vi "LV_UDP_client.vi"() -> ()   [LabVIEW 2020]
panel:
  in  "Send Test Image":bool
  in  "h":i32=10 min=1 max=5000 step=1
  in  "w":i32=1 min=1 max=5000 step=1
  out "Elaps ms":u32
  in  "Send Image":bool
  out "Path to Python script":path
  in  "Stop":bool
  out "Answer":string
  in  "Ping":bool
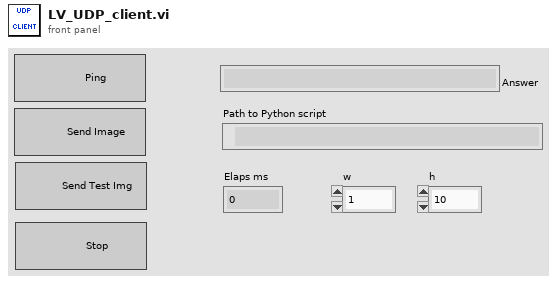
[diagram p1: front panel]
types:
  T1 = typedef "Image Type" = u32
  T2 = enum8{"Enabled", "Disabled", "Disabled and Grayed Out"}
  T3 = typedef "IMAQ Image.ctl" = refnum<image>
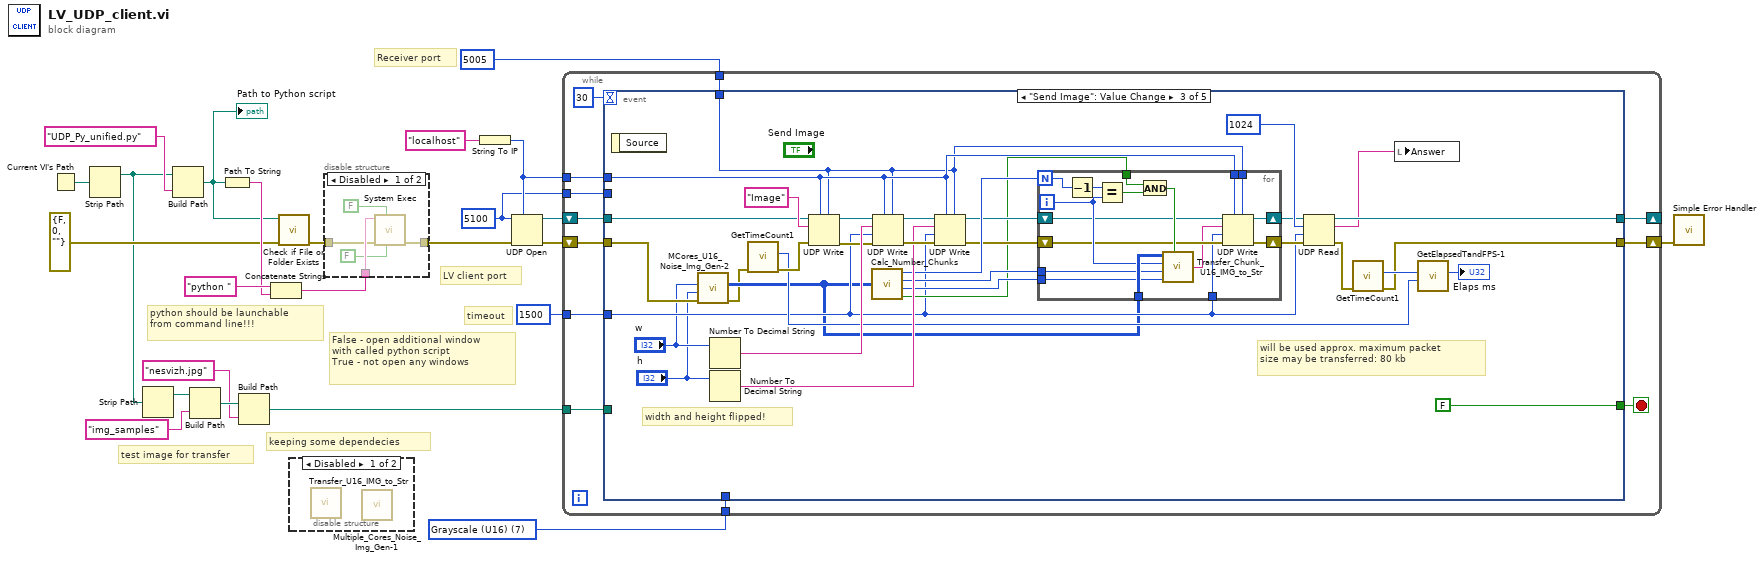
[diagram p0: block diagram]
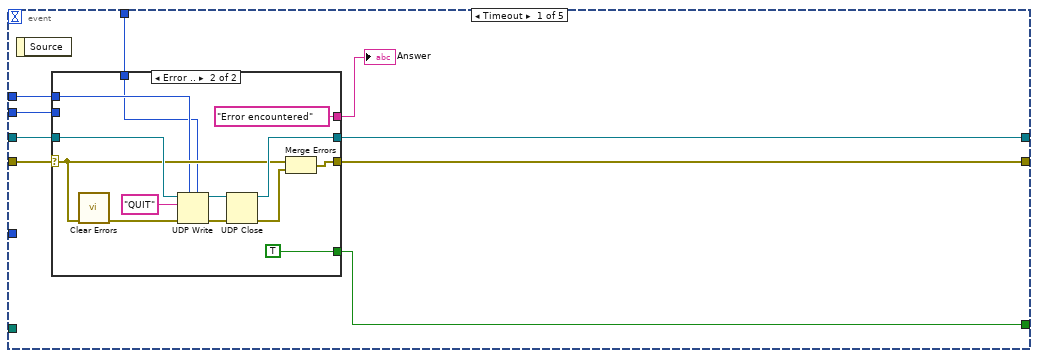
[diagram p4: hidden frame]
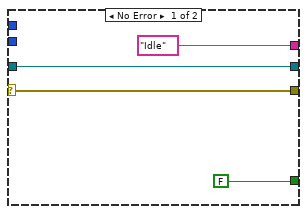
[diagram p5: hidden frame]
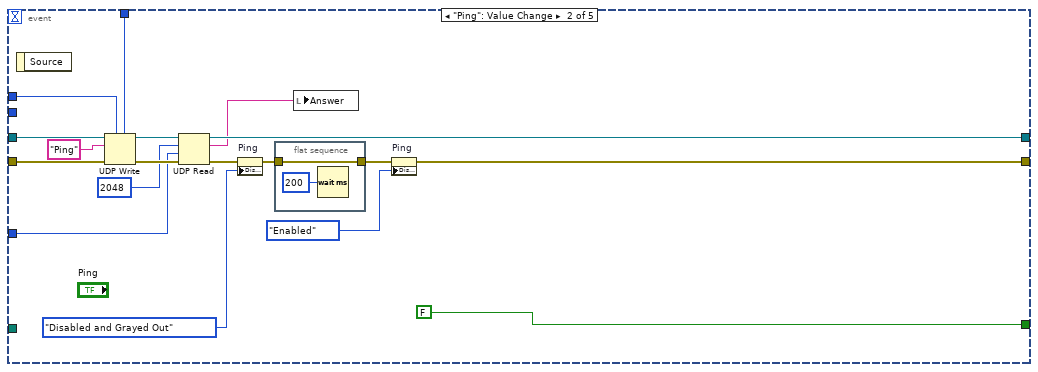
[diagram p6: hidden frame]
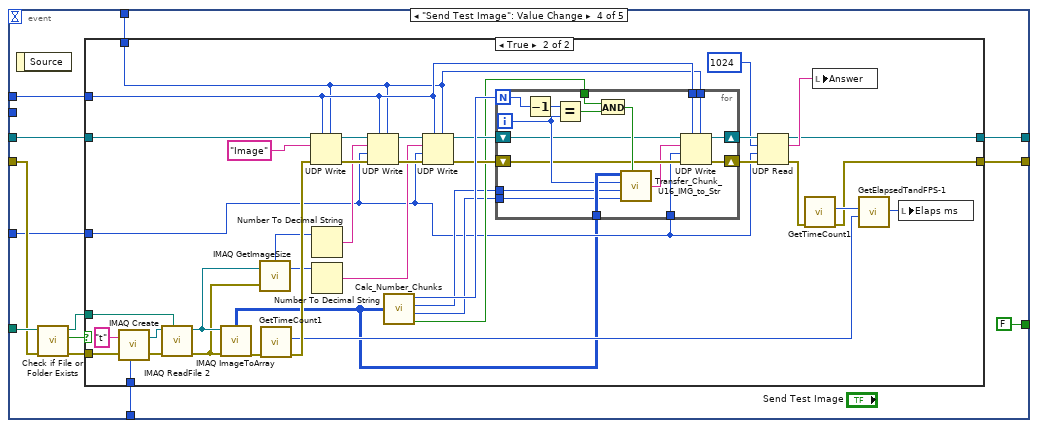
[diagram p7: hidden frame]
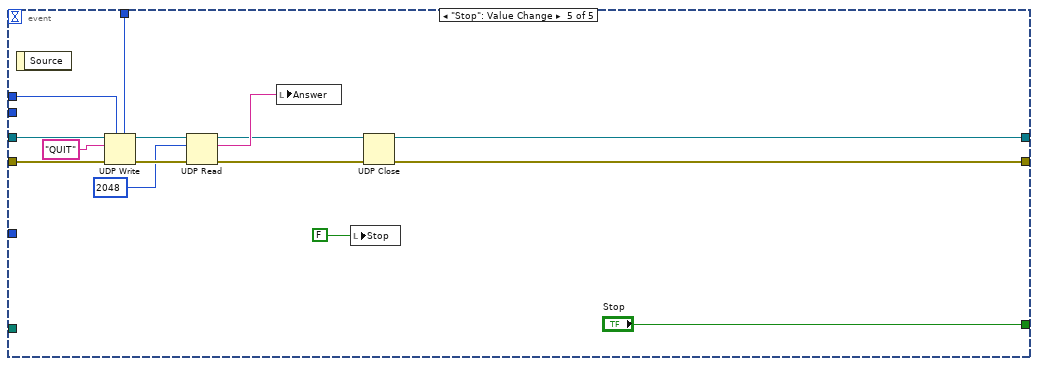
[diagram p9: hidden frame]
diagram:
  w1 = T1 7 items=["Grayscale (U8)", "Grayscale (I16)", "Grayscale (SGL)", "Complex (CSG)", "RGB (U32)", "HSL (U32)", "RGB (U64)", "Grayscale (U16)"] ("Image Type")
  w10 = u16 5100 ("remote port or service name")
  # "test image for transfer"
  # "keeping some dependecies"
  # "timeout"
  # "Receiver port"
  # "LV client port"
  # "False - open additional window\nwith called python script\nTrue - not open any windows"
  # "python should be launchable \nfrom command line!!!"
  n1 = Current VI's Path() -> (path=w23:path)
  n2 = Strip Path(path=w23) -> (stripped path=w7:path)  [unwired: 1 out]
  n3 = Strip Path(path=w7) -> (stripped path=w6:path)  [unwired: 1 out]
  n4 = Build Path(base path=w7, name or relative path="UDP_Py_unified.py" ("string")) -> (appended path=w17:path)
  "Path to Python script" <- w17
  n5 = Build Path(base path=w6, name or relative path="img_samples" ("string")) -> (appended path=w4:path)
  n6 = Path To String(path=w17) -> (string=w19:string)
  n7 = Build Path(base path=w4, name or relative path="nesvizh.jpg" ("string")) -> (appended path=w2:path)
  n8 = Concatenate Strings("python " ("command line"), w19) -> (w21:string)
  n9 = call <vilib>:"Check if File or Folder Exists.vi"("error in (no error)"=errorcluster {"status"=FALSE, "code"=0, "source"=""}, "path"=w17) -> ("error out"=w16:errorcluster)  [unwired: 7 in, 2 out]
  n10 = disable-structure shown="Disabled" {
    frame Disabled {
      n11 = call "Transfer_U16_IMG_to_Str.vi"() -> ()  [unwired: 1 in, 1 out]
      n12 = call "Multiple_Cores_Noise_Img_Gen-1.vi"() -> ()  [unwired: 10 in, 2 out]
    }
    frame Enabled {
    }
  }
  n13 = disable-structure shown="Disabled" {
    disable-tunnel: w21 -> [w29 _]
    disable-tunnel: [w28 w30] -> w15
    disable-tunnel: w16 -> [w26 w30]
    frame Disabled {
      n14 = call <vilib>:"System Exec.vi"("run minimized? (F)"=FALSE, "wait until completion? (T)"=FALSE, "error in (no error)"=w26, "command line"=w29) -> ("error out"=w28:errorcluster)  [unwired: 4 in, 3 out]
    }
    frame Enabled {
    }
  }
  n15 = String To IP(1:"localhost" ("address")) -> (0:w11:u32)
  n16 = UDP Open(7:w11, 8:w15, 11:w10) -> (port=w13:refnum<k16>, 0:w14:errorcluster)  [unwired: 2 in, 1 out]
  n17 = while {
    shift-right: [w39] -> _
    shift-left: w13 -> [w40]
    shift-right: [w37] -> w24
    shift-left: w14 -> [w41]
    tunnel: w11 -> [w35]
    tunnel: w10 -> [w36]
    tunnel: u16 5005 ("remote port or service name") -> [w34]
    tunnel: 1500 -> [w33]
    tunnel: w2 -> [w32]
    tunnel: w1 -> [w31]
    stop <- w38 stop-if-true
    n18 = event shown="[2] \"Send Image\": Value Change" {
      selector: _ -> [_ _ _ _ _]
      dyn-events: _ -> [_ _ _ _ _]
      timeout: 30 -> [_ _ _ _ _]
      tunnel: [w47 FALSE ("Stop") FALSE ("Stop") FALSE ("Stop") "Stop"] -> w38
      tunnel: w41 -> [w51 w80 w93 w150 w221]
      tunnel: w40 -> [w50 w79 w121 w145 w222]
      tunnel: [w49 w75 w115 w140 w223] -> w39
      tunnel: [w48 w82 w106 w141 w224] -> w37
      tunnel: w36 -> [w45 _ _ _ _]
      tunnel: w35 -> [w44 w71 w95 w144 w213]
      tunnel: w34 -> [w43 w70 w94 w143 w212]
      tunnel: w33 -> [_ w69 w96 w142 _]
      tunnel: w32 -> [_ _ _ w151 _]
      tunnel: w31 -> [_ _ _ w146 _]
      event Timeout {
        n19 = event-data() -> ()  [unwired: 1 in, 1 out]
        n20 = case shown="Error .." w51 {
          selector: w51 -> [w54 w59]
          tunnel: [w55 w66] -> w49
          tunnel: w50 -> [w55 w65]
          tunnel: [w54 w60] -> w48
          tunnel: [FALSE ("Stop") TRUE ("Stop")] -> w47
          tunnel: ["Idle" ("Answer") "Error encountered" ("Answer")] -> w46
          tunnel: w45 -> [_ _]
          tunnel: w44 -> [_ w57]
          tunnel: w43 -> [_ w56]
          frame No Error {
          }
          frame Error {
            n21 = call <vilib>:"Clear Errors.vi"("error in (no error)"=w59) -> ("error out"=w64:errorcluster)  [unwired: 5 in, 1 out]
            n22 = UDP Write(address=w57, port or service name=w56, connection ID=w65, data in="QUIT", 8:w64) -> (error out=w63:errorcluster, 3:w61:refnum<k16>)  [unwired: 1 in]
            n23 = UDP Close(connection ID=w61, 8:w63) -> (connection ID out=w66:refnum<k16>, error out=w58:errorcluster)
            n24 = Merge Errors(w59, w58) -> (w60:errorcluster)
          }
        }
        "Answer" <- w46
      }
      event "Ping": Value Change {
        n25 = event-data() -> ()  [unwired: 1 in, 1 out]
        n26 = UDP Write(address=w71, port or service name=w70, connection ID=w79, data in="Ping", 8:w80) -> (error out=w77:errorcluster, 3:w76:refnum<k16>)  [unwired: 1 in]
        n27 = UDP Read(connection ID=w76, max size (548)=2048 ("bytes to read"), timeout ms (25000)=w69, 8:w77) -> (data out=w72:string, error out=w74:errorcluster, 3:w75:refnum<k16>)  [unwired: 2 out]
        n28 = property on="Ping" class="Bool"(error in=w74, "DisabledEnum"=T2."Disabled and Grayed Out" ("Disabled")) -> (error out=w85:errorcluster)  [unwired: 1 in, 1 out]
        n29 = flat-sequence {
          tunnel: w85 -> [w87]
          tunnel: [w87] -> w83
          frame #0 {
            n30 = Wait (ms)(milliseconds to wait=u32 200) -> ()  [unwired: 1 out]
          }
        }
        n31 = local write "Answer"(w72) -> ()
        n32 = property on="Ping" class="Bool"(error in=w83, "DisabledEnum"=T2."Enabled" ("Disabled")) -> (error out=w82:errorcluster)  [unwired: 1 in, 1 out]
      }
      event "Send Image": Value Change {
        # "width and height flipped!"
        # "will be used approx. maximum packet \nsize may be transferred: 80 kb"
        n33 = event-data() -> ()  [unwired: 1 in, 1 out]
        n34 = call "MCores_U16_Noise_Img_Gen-2.vi"("error IN"=w93, "[IN] Width"="h", "[IN] Height"="w") -> ("error OUT"=w91:errorcluster, "[OUT] U16 Pixel Img"=w92:u16[][])  [unwired: 7 in]
        n35 = Number To Decimal String(number="w") -> (decimal integer string=w117:string)  [unwired: 1 in]
        n36 = Number To Decimal String(number="h") -> (decimal integer string=w113:string)  [unwired: 1 in]
        n37 = call "GetTimeCount1.vi"("error IN"=w91) -> ("error OUT"=w110:errorcluster, "[OUT] Timer Count"=w107:u32)  [unwired: 9 in]
        n38 = UDP Write(address=w95, port or service name=w94, connection ID=w121, data in="Image", 8:w110) -> (error out=w111:errorcluster, 3:w112:refnum<k16>)  [unwired: 1 in]
        n39 = call "Calc_Number_Chunks.vi"("[IN] U16 Pixel Img"=w92) -> ("[OUT] Number of chunks"=w103:i32, "[OUT] # rows single transfer"=w102:i32, "[OUT] # rows last transfer"=w101:i32, "[OUT] Not-equal last transfer"=w97:bool)
        n40 = UDP Write(address=w95, port or service name=w94, connection ID=w112, data in=w117, 8:w111, 9:w96) -> (error out=w120:errorcluster, 3:w119:refnum<k16>)
        n41 = UDP Write(address=w95, port or service name=w94, connection ID=w119, data in=w113, 8:w120, 9:w96) -> (error out=w99:errorcluster, 3:w100:refnum<k16>)
        n42 = for {
          N: w103 -> [w139]
          shift-right: [w129] -> w104
          shift-left: w99 -> [w130]
          tunnel: w92 -> [w137]
          tunnel: w102 -> [w132]
          tunnel: w101 -> [w131]
          shift-right: [w128] -> w98
          shift-left: w100 -> [w127]
          tunnel: w97 -> [w134]
          tunnel: w96 -> [w125]
          tunnel: w95 -> [w124]
          tunnel: w94 -> [w123]
          i -> [w135]
          n43 = Decrement(x=w139) -> (x-1=w138:i32)
          n44 = Equal?(x=w138, y=w135) -> (x = y?=w133:bool)
          n45 = And(x=w134, y=w133) -> (x .and. y?=w136:bool)
          n46 = call "Transfer_Chunk_U16_IMG_to_Str.vi"("[IN] U16 Pixel Img"=w137, "[IN] # of chunk"=w135, "[IN] # rows single transfer"=w132, "[IN] # rows last transfer"=w131, "[IN] Use remained rows"=w136) -> ("[OUT] Converted String"=w126:string)
          n47 = UDP Write(address=w124, port or service name=w123, connection ID=w127, data in=w126, 8:w130, 9:w125) -> (error out=w129:errorcluster, 3:w128:refnum<k16>)
        }
        n48 = UDP Read(connection ID=w98, max size (548)=1024 ("bytes to read"), timeout ms (25000)=w96, 8:w104) -> (data out=w114:string, error out=w109:errorcluster, 3:w115:refnum<k16>)  [unwired: 2 out]
        n49 = call "GetTimeCount1.vi"("error IN"=w109) -> ("error OUT"=w106:errorcluster, "[OUT] Timer Count"=w108:u32)  [unwired: 9 in]
        n50 = local write "Answer"(w114) -> ()
        n51 = call "GetElapsedTandFPS-1.vi"("[IN] Timer Count Before ALL [ms]"=w107, "[IN] Timer Count After ALL [ms]"=w108) -> ("[OUT] Elapsed time [ms]"=→"Elaps ms":u32)  [unwired: 3 in, 2 out]
      }
      event "Send Test Image": Value Change {
        n52 = event-data() -> ()  [unwired: 1 in, 1 out]
        n53 = call <vilib>:"Check if File or Folder Exists.vi"("error in (no error)"=w150, "path"=w151) -> ("error out"=w149:errorcluster, "file or folder exists?"=w148:bool, "dup path"=w147:path)  [unwired: 7 in]
        n54 = case shown="True" w148 {
          tunnel: w149 -> [w153 w194]
          tunnel: w147 -> [_ w189]
          tunnel: w146 -> [_ w193]
          tunnel: w145 -> [w154 w187]
          tunnel: w144 -> [_ w168]
          tunnel: w143 -> [_ w167]
          tunnel: w142 -> [_ w164]
          tunnel: [w153 w157] -> w141
          tunnel: [w154 w156] -> w140
          frame False {
          }
          frame True {
            n55 = call "IMAQ Create"("Image Name"="t", "Image Type"=w193, "error in (no error)"=w194) -> ("New Image"=w190:T3, "error out"=w191:errorcluster)  [unwired: 2 in]
            n56 = call "IMAQ ReadFile 2"("File Path"=w189, "error in (no error)"=w191, "Image"=w190) -> ("error out"=w183:errorcluster, "Image Out"=w184:T3)  [unwired: 4 in, 3 out]
            n57 = call "IMAQ ImageToArray"("error in (no error)"=w183, "Image"=w184) -> ("error out"=w188:errorcluster, "Image Pixels (U8)"=w155:u8[][])  [unwired: 2 in, 3 out]
            n58 = call "IMAQ GetImageSize"("Image"=w184, "error in (no error)"=w183) -> ("Y Resolution"=w181:i32, "X Resolution"=w182:i32)  [unwired: 2 in, 1 out]
            n59 = call "GetTimeCount1.vi"("error IN"=w188) -> ("error OUT"=w186:errorcluster, "[OUT] Timer Count"=w160:u32)  [unwired: 9 in]
            n60 = UDP Write(address=w168, port or service name=w167, connection ID=w187, data in="Image", 8:w186) -> (error out=w180:errorcluster, 3:w179:refnum<k16>)  [unwired: 1 in]
            n61 = Number To Decimal String(number=w182) -> (decimal integer string=w178:string)  [unwired: 1 in]
            n62 = Number To Decimal String(number=w181) -> (decimal integer string=w175:string)  [unwired: 1 in]
            n63 = UDP Write(address=w168, port or service name=w167, connection ID=w179, data in=w178, 8:w180, 9:w164) -> (error out=w176:errorcluster, 3:w177:refnum<k16>)
            n64 = call "Calc_Number_Chunks.vi"("[IN] U16 Pixel Img"=w155) -> ("[OUT] Number of chunks"=w174:i32, "[OUT] # rows single transfer"=w170:i32, "[OUT] # rows last transfer"=w169:i32, "[OUT] Not-equal last transfer"=w171:bool)
            n65 = UDP Write(address=w168, port or service name=w167, connection ID=w177, data in=w175, 8:w176, 9:w164) -> (error out=w172:errorcluster, 3:w173:refnum<k16>)
            n66 = for {
              N: w174 -> [w211]
              shift-right: [w201] -> w166
              shift-left: w172 -> [w202]
              tunnel: w155 -> [w209]
              tunnel: w170 -> [w204]
              tunnel: w169 -> [w203]
              shift-right: [w200] -> w165
              shift-left: w173 -> [w199]
              tunnel: w171 -> [w206]
              tunnel: w164 -> [w197]
              tunnel: w168 -> [w196]
              tunnel: w167 -> [w195]
              i -> [w207]
              n67 = Decrement(x=w211) -> (x-1=w210:i32)
              n68 = Equal?(x=w210, y=w207) -> (x = y?=w205:bool)
              n69 = And(x=w206, y=w205) -> (x .and. y?=w208:bool)
              n70 = call "Transfer_Chunk_U16_IMG_to_Str.vi"("[IN] U16 Pixel Img"=w209, "[IN] # of chunk"=w207, "[IN] # rows single transfer"=w204, "[IN] # rows last transfer"=w203, "[IN] Use remained rows"=w208) -> ("[OUT] Converted String"=w198:string)
              n71 = UDP Write(address=w196, port or service name=w195, connection ID=w199, data in=w198, 8:w202, 9:w197) -> (error out=w201:errorcluster, 3:w200:refnum<k16>)
            }
            n72 = UDP Read(connection ID=w165, max size (548)=1024 ("bytes to read"), timeout ms (25000)=w164, 8:w166) -> (data out=w163:string, error out=w162:errorcluster, 3:w156:refnum<k16>)  [unwired: 2 out]
            n73 = call "GetTimeCount1.vi"("error IN"=w162) -> ("error OUT"=w157:errorcluster, "[OUT] Timer Count"=w161:u32)  [unwired: 9 in]
            n74 = local write "Answer"(w163) -> ()
            n75 = call "GetElapsedTandFPS-1.vi"("[IN] Timer Count Before ALL [ms]"=w160, "[IN] Timer Count After ALL [ms]"=w161) -> ("[OUT] Elapsed time [ms]"=w158:u32)  [unwired: 3 in, 2 out]
            n76 = local write "Elaps ms"(w158) -> ()
          }
        }
      }
      event "Stop": Value Change {
        n77 = event-data() -> ()  [unwired: 1 in, 1 out]
        n78 = UDP Write(address=w213, port or service name=w212, connection ID=w222, data in="QUIT", 8:w221) -> (error out=w218:errorcluster, 3:w219:refnum<k16>)  [unwired: 1 in]
        n79 = UDP Read(connection ID=w219, max size (548)=2048 ("bytes to read"), 8:w218) -> (data out=w216:string, error out=w217:errorcluster, 3:w215:refnum<k16>)  [unwired: 1 in, 2 out]
        n80 = local write "Answer"(w216) -> ()
        n81 = local write "Stop"(FALSE ("Stop")) -> ()
        n82 = UDP Close(connection ID=w215, 8:w217) -> (connection ID out=w223:refnum<k16>, error out=w224:errorcluster)
      }
    }
  }
  n83 = call <vilib>:"Simple Error Handler.vi"("error in (no error)"=w24) -> ()  [unwired: 4 in, 5 out]
